vi "ToRepo.vi"(8 "error in":errorcluster, 9 "to repo cluster":T1, 10 "repository in":refnum<class "NISE_CEF_Repository.lvclass">, 11 "engine in":refnum<class "Engine Parent Editor Node.lvclass">) -> (0 "error out":errorcluster, 2 "repository out":refnum<class "NISE_CEF_Repository.lvclass">, 3 "Engine out":refnum<class "Engine Parent Editor Node.lvclass">)   [LabVIEW 2013, in "PL Framework Configuration Tool.lvlib" / "Engine Parent Editor Node.lvclass"]
doc: "Transfers the information from the tree node into the repo. How it is stored in the repo depends on the Repo."
uses:
  Engine Parent Editor Node.lvclass
  <vilib>/NI/Configuration Framework/Repository/NISE_CEF_Repository.lvclass
  <vilib>/NI/Configuration Framework/Node/ToRepoCluster.ctl
  SystemConfigRepo/SystemConfigRepo.lvclass
  to repo data.ctl
  Module editor node/to repo data.ctl
  SystemConfigRepo/SystemConfigRepo.lvclass/SystemConfigRepo.ctl
  TBM Configuration Node/TBM Configuration Node.lvclass
  Framework Configuration Classes/platypus configuration/engines cluster.ctl
  <vilib>/NI/Module Execution Interface/Engine Configuration/engine configuration.lvclass
  <vilib>/NI/Tag Bus Module Framework/module configuration/TBM module configuration.lvclass
  Module editor node/module editor node.lvclass
  <vilib>/NI/Configuration Framework/Node/NISE_CEF_Node.lvclass
  Framework Configuration Classes/platypus configuration/PLConfigurationSerializer.lvlib
  <vilib>/NI/Configuration Framework/serializable configuration/NISE_CEF_serializable configuration.lvclass
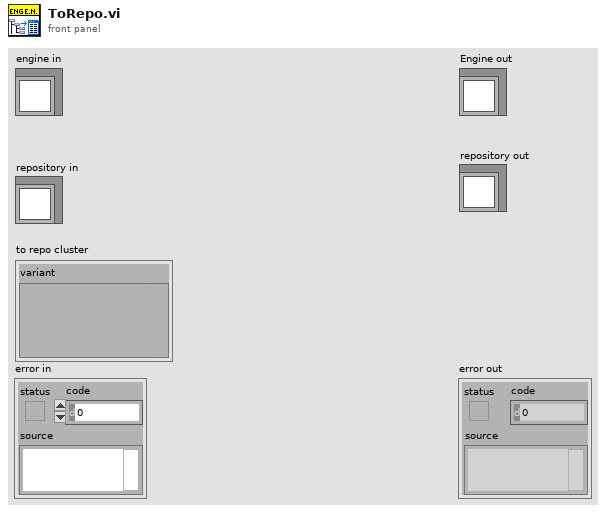
[diagram p1: front panel]
types:
  T1 = typedef "NISE_CEF_Node.lvclass/ToRepoCluster.ctl" = cluster{"variant":variant}
  T2 = typedef "PL Framework Configuration Tool.lvlib/module editor node.lvclass/to repo data.ctl" = cluster{"target index":i32, "engine index":i32}
  T3 = typedef "PL Framework Configuration Tool.lvlib/Engine Parent Editor Node.lvclass/to repo data.ctl" = cluster{"target index":i32}
  T4 = typedef "PLConfigurationSerializer.lvlib/targets cluster.ctl" = cluster{"Target Configuration":refnum<class "PL_Target Configuration.lvclass">, "engines":T5[]}
  T5 = typedef "PLConfigurationSerializer.lvlib/engines cluster.ctl" = cluster{"engine configuration":refnum<class "engine configuration.lvclass">, "modules":refnum<class "TBM module configuration.lvclass">[]}
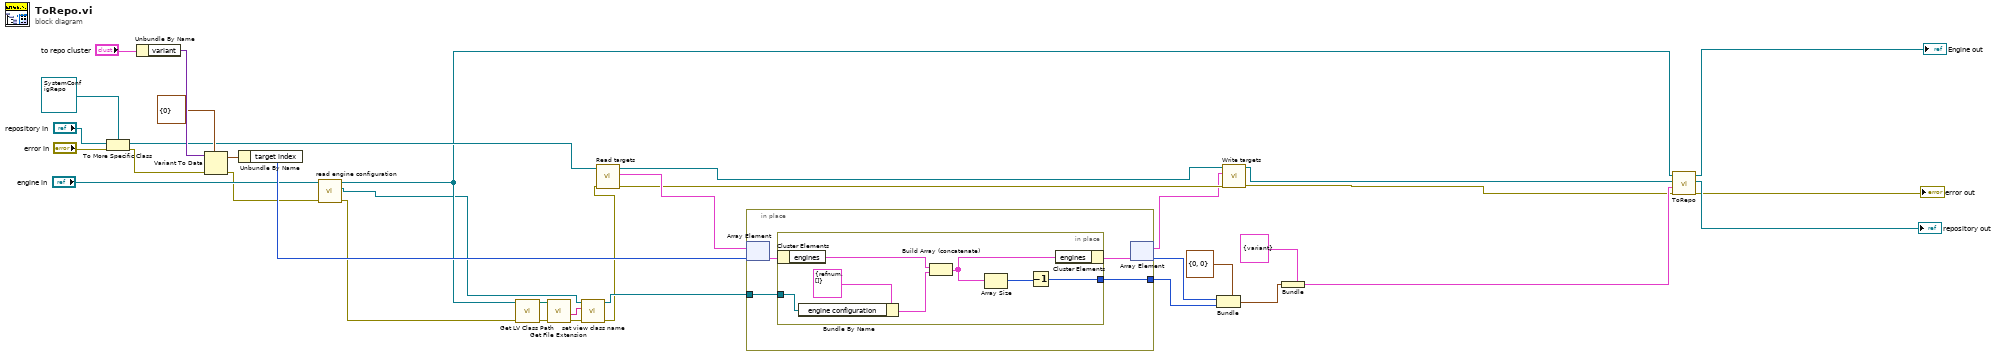
[diagram p0: block diagram]
diagram:
  n1 = To More Specific Class(target class=refnum<class "SystemConfigRepo.lvclass"> refnum ("SystemConfigRepo.lvclass"), reference="repository in", error in="error in") -> (specific class reference=w16:refnum<class "SystemConfigRepo.lvclass">, error out=w33:errorcluster)
  n2 = Unbundle By Name("to repo cluster") -> ("variant"=w31:variant)
  n3 = Variant To Data(error in=w33, type=T3 {"target index"=0} ("to repo data"), Variant=w31) -> (data=w29:T3, error out=w17:errorcluster)
  n4 = Unbundle By Name(w29) -> ("target index"=w28:i32)
  n5 = call "read engine configuration.vi"("error in"=w17, "Engine Parent Editor Node in"="engine in") -> ("error out"=w2:errorcluster, "engine configuration"=w4:refnum<class "engine configuration.lvclass">, "Engine Parent Editor Node out"=w5:refnum<class "Engine Parent Editor Node.lvclass">)  [unwired: 7 in]
  n6 = call <vilib>:"Get LV Class Path.vi"("error in (no error)"=w2, "object"=w5) -> ("error out"=w9:errorcluster, "class path"=w8:path)  [unwired: 8 in]
  n7 = call <vilib>:"Get File Extension.vi"("error in (no error)"=w9, "file"=w8) -> ("error out"=w7:errorcluster, "filename without extension"=w6:string)  [unwired: 6 in, 2 out]
  n8 = call <vilib>:"set view class name.vi"("error in"=w7, "view class"=w6, "configuration in"=w4) -> ("error out"=w1:errorcluster, "configuration out"=w3:refnum<class "engine configuration.lvclass">)  [unwired: 7 in]
  n9 = call "Read targets.vi"("error in"=w1, "SystemConfigRepo in"=w16) -> ("error out"=w14:errorcluster, "targets"=w15:T4[], "SystemConfigRepo out"=w12:refnum<class "SystemConfigRepo.lvclass">)  [unwired: 7 in]
  n10 = in-place {
    in-place-border: w3 -> [w38]
    in-place-border: [w37] -> w24
    n11 = in-place-array #1(w15, w28) -> (w40:T4)
    n12 = in-place {
      in-place-border: w38 -> [w46]
      in-place-border: [w41] -> w37
      n13 = in-place-cluster #2(w40) -> ("engines"=w45:T5[])
      n14 = Bundle By Name(cluster=T5 {"engine configuration"=refnum, "modules"=[]} ("engines cluster"), "engine configuration"=w46) -> (w44:T5)
      n15 = Build Array (concatenate)(w45, w44) -> (w43:T5[])
      n16 = Array Size(array=w43) -> (size(s)=w42:i32)
      n17 = Decrement(x=w42) -> (x-1=w41:i32)
      n18 = in-place-cluster #2("engines"=w43) -> (w39:T4)
    }
    n19 = in-place-array #1(w39) -> (w13:T4[], w23:i32)
  }
  n20 = Bundle(cluster=T2 {"target index"=0, "engine index"=0} ("to repo data"), "target index"=w23, "engine index"=w24) -> (w25:T2)
  n21 = call "Write targets.vi"("error in"=w14, "targets"=w13, "SystemConfigRepo in"=w12) -> ("error out"=w11:errorcluster, "SystemConfigRepo out"=w10:refnum<class "SystemConfigRepo.lvclass">)  [unwired: 7 in]
  n22 = Bundle(cluster=T1 {"variant"=variant} ("to repo cluster"), "variant"=w25) -> (w19:T1)
  n23 = call-parent "ToRepo.vi"("error in"=w11, "to repo cluster"=w19, "repository in"=w10, "node in"=w5) -> ("error out"=→"error out":errorcluster, "repository out"=→"repository out":refnum<class "NISE_CEF_Repository.lvclass">, "node out"=→"Engine out":refnum<class "Engine Parent Editor Node.lvclass">)  [unwired: 5 in]
